vi "Periodic String Filter2.vi"(0 "Input String":string, 1 "reset?":bool, 2 "State":T1, 5 "Parameter":string, 9 "Remove Immediately?(F)":bool, 11 "Settings":T2={"threashold(#/s)"=1.0, "Check Peroid(s)"=1.0}, 12 "Exceeding processing capacity(F)":bool) -> (4 "Input String(dup)":string, 6 "oper":string, 8 ">> String-Parameter Map >>":variant=variant("CSM Tiny.DAQ: Break Continuous"=variant(u32 953145328), "CSM Tiny.DAQ: Close"=variant(u32 953145328), "CSM Tiny.DAQ: Configure"=variant(u32 953126122), "CSM Tiny.DAQ: Continuous Check"=variant(u32 953144928), "CSM Tiny.DAQ: Initialize"=variant(u32 953126122), "CSM Tiny.DAQ: Start"=variant(u32 953126122), "CSM Tiny.DAQ: Stop"=variant(u32 953145328), "CSM Tiny.Data"=variant(u32 953144928), "CSM Tiny.Data: Acquisite"=variant(u32 953144928), "CSM Tiny.UI: Refresh Buttons"=variant(u32 953145328)), 10 "Filtered Status":T3[](array[typedef]), 13 "Info":string[](array[string]), 14 "removed info":T3[](array[typedef]), 15 "filtered?":bool)   [LabVIEW 2017]
uses:
  user.lib/_NEVSTOP/Communicable State Machine(CSM)/Utility/Periodic String Filter Info.ctl
  user.lib/_NEVSTOP/Communicable State Machine(CSM)/Utility/Periodic String Filter State.ctl
  user.lib/_NEVSTOP/Communicable State Machine(CSM)/Communicable State Machine.lvlib
panel:
  out ">> Log Last Update Timestamp Map >>":variant=variant("CSM Tiny.DAQ: Break Continuous"=variant(u32 953145328), "CSM Tiny.DAQ: Close"=variant(u32 953145328), "CSM Tiny.DAQ: Configure"=variant(u32 953126122), "CSM Tiny.DAQ: Continuous Check"=variant(u32 953144928), "CSM Tiny.DAQ: Initialize"=variant(u32 953126122), "CSM Tiny.DAQ: Start"=variant(u32 953126122), "CSM Tiny.DAQ: Stop"=variant(u32 953145328), "CSM Tiny.Data"=variant(u32 953144928), "CSM Tiny.Data: Acquisite"=variant(u32 953144928), "CSM Tiny.UI: Refresh Buttons"=variant(u32 953145328))
  out ">> Log Count Map >>":variant=variant("CSM Tiny.DAQ: Break Continuous"=variant(i64 1), "CSM Tiny.DAQ: Close"=variant(i64 1), "CSM Tiny.DAQ: Configure"=variant(i64 1), "CSM Tiny.DAQ: Continuous Check"=variant(i64 192), "CSM Tiny.DAQ: Initialize"=variant(i64 1), "CSM Tiny.DAQ: Start"=variant(i64 1), "CSM Tiny.DAQ: Stop"=variant(i64 1), "CSM Tiny.Data"=variant(i64 97), "CSM Tiny.Data: Acquisite"=variant(i64 97), "CSM Tiny.UI: Refresh Buttons"=variant(i64 3))
  out ">> Log Last Check Count Map >>":variant=variant("CSM Tiny.DAQ: Break Continuous"=variant(i64 1), "CSM Tiny.DAQ: Close"=variant(i64 1), "CSM Tiny.DAQ: Configure"=variant(i64 1), "CSM Tiny.DAQ: Continuous Check"=variant(i64 188), "CSM Tiny.DAQ: Initialize"=variant(i64 1), "CSM Tiny.DAQ: Start"=variant(i64 1), "CSM Tiny.DAQ: Stop"=variant(i64 1), "CSM Tiny.Data"=variant(i64 95), "CSM Tiny.Data: Acquisite"=variant(i64 95), "CSM Tiny.UI: Refresh Buttons"=variant(i64 2))
  out ">> Log Last Check Timestamp Map >>":variant=variant("CSM Tiny.DAQ: Break Continuous"=variant(u32 953145328), "CSM Tiny.DAQ: Close"=variant(u32 953145328), "CSM Tiny.DAQ: Configure"=variant(u32 953126122), "CSM Tiny.DAQ: Continuous Check"=variant(u32 953144928), "CSM Tiny.DAQ: Initialize"=variant(u32 953126122), "CSM Tiny.DAQ: Start"=variant(u32 953126122), "CSM Tiny.DAQ: Stop"=variant(u32 953145328), "CSM Tiny.Data"=variant(u32 953144928), "CSM Tiny.Data: Acquisite"=variant(u32 953144928), "CSM Tiny.UI: Refresh Buttons"=variant(u32 953145328))
  out ">> Filtered Log Count Map >>":variant=variant("CSM Tiny.DAQ: Break Continuous"=variant(i64 1), "CSM Tiny.DAQ: Close"=variant(i64 1), "CSM Tiny.DAQ: Configure"=variant(i64 1), "CSM Tiny.DAQ: Continuous Check"=variant(i64 188), "CSM Tiny.DAQ: Initialize"=variant(i64 1), "CSM Tiny.DAQ: Start"=variant(i64 1), "CSM Tiny.DAQ: Stop"=variant(i64 1), "CSM Tiny.Data"=variant(i64 95), "CSM Tiny.Data: Acquisite"=variant(i64 95), "CSM Tiny.UI: Refresh Buttons"=variant(i64 2))
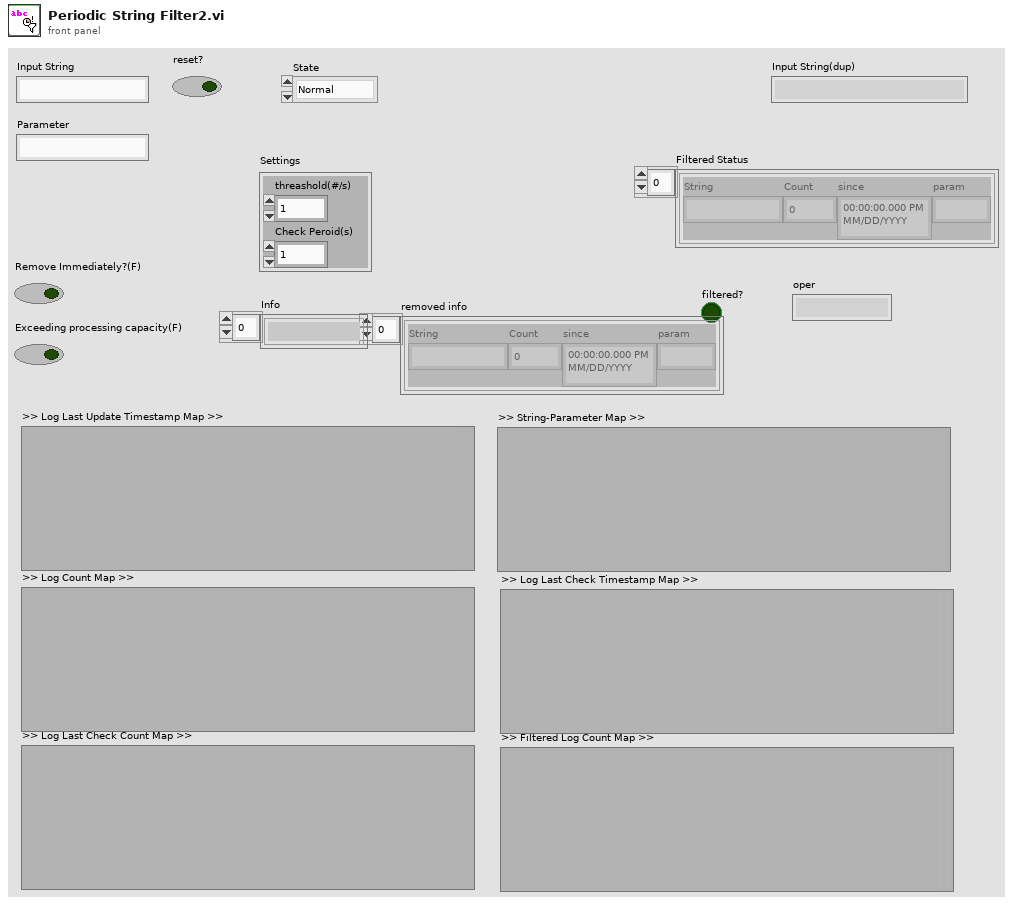
[diagram p1: front panel]
types:
  T1 = typedef "Communicable State Machine.lvlib/Periodic String Filter State.ctl" = enum16{"Normal", "Remove All Filters"}
  T2 = cluster{"threashold(#/s)":dbl, "Check Peroid(s)":dbl}
  T3 = typedef "Communicable State Machine.lvlib/Periodic String Filter Info.ctl" = cluster{"String":string, "Count":i64, "since":timestamp, "param":string}
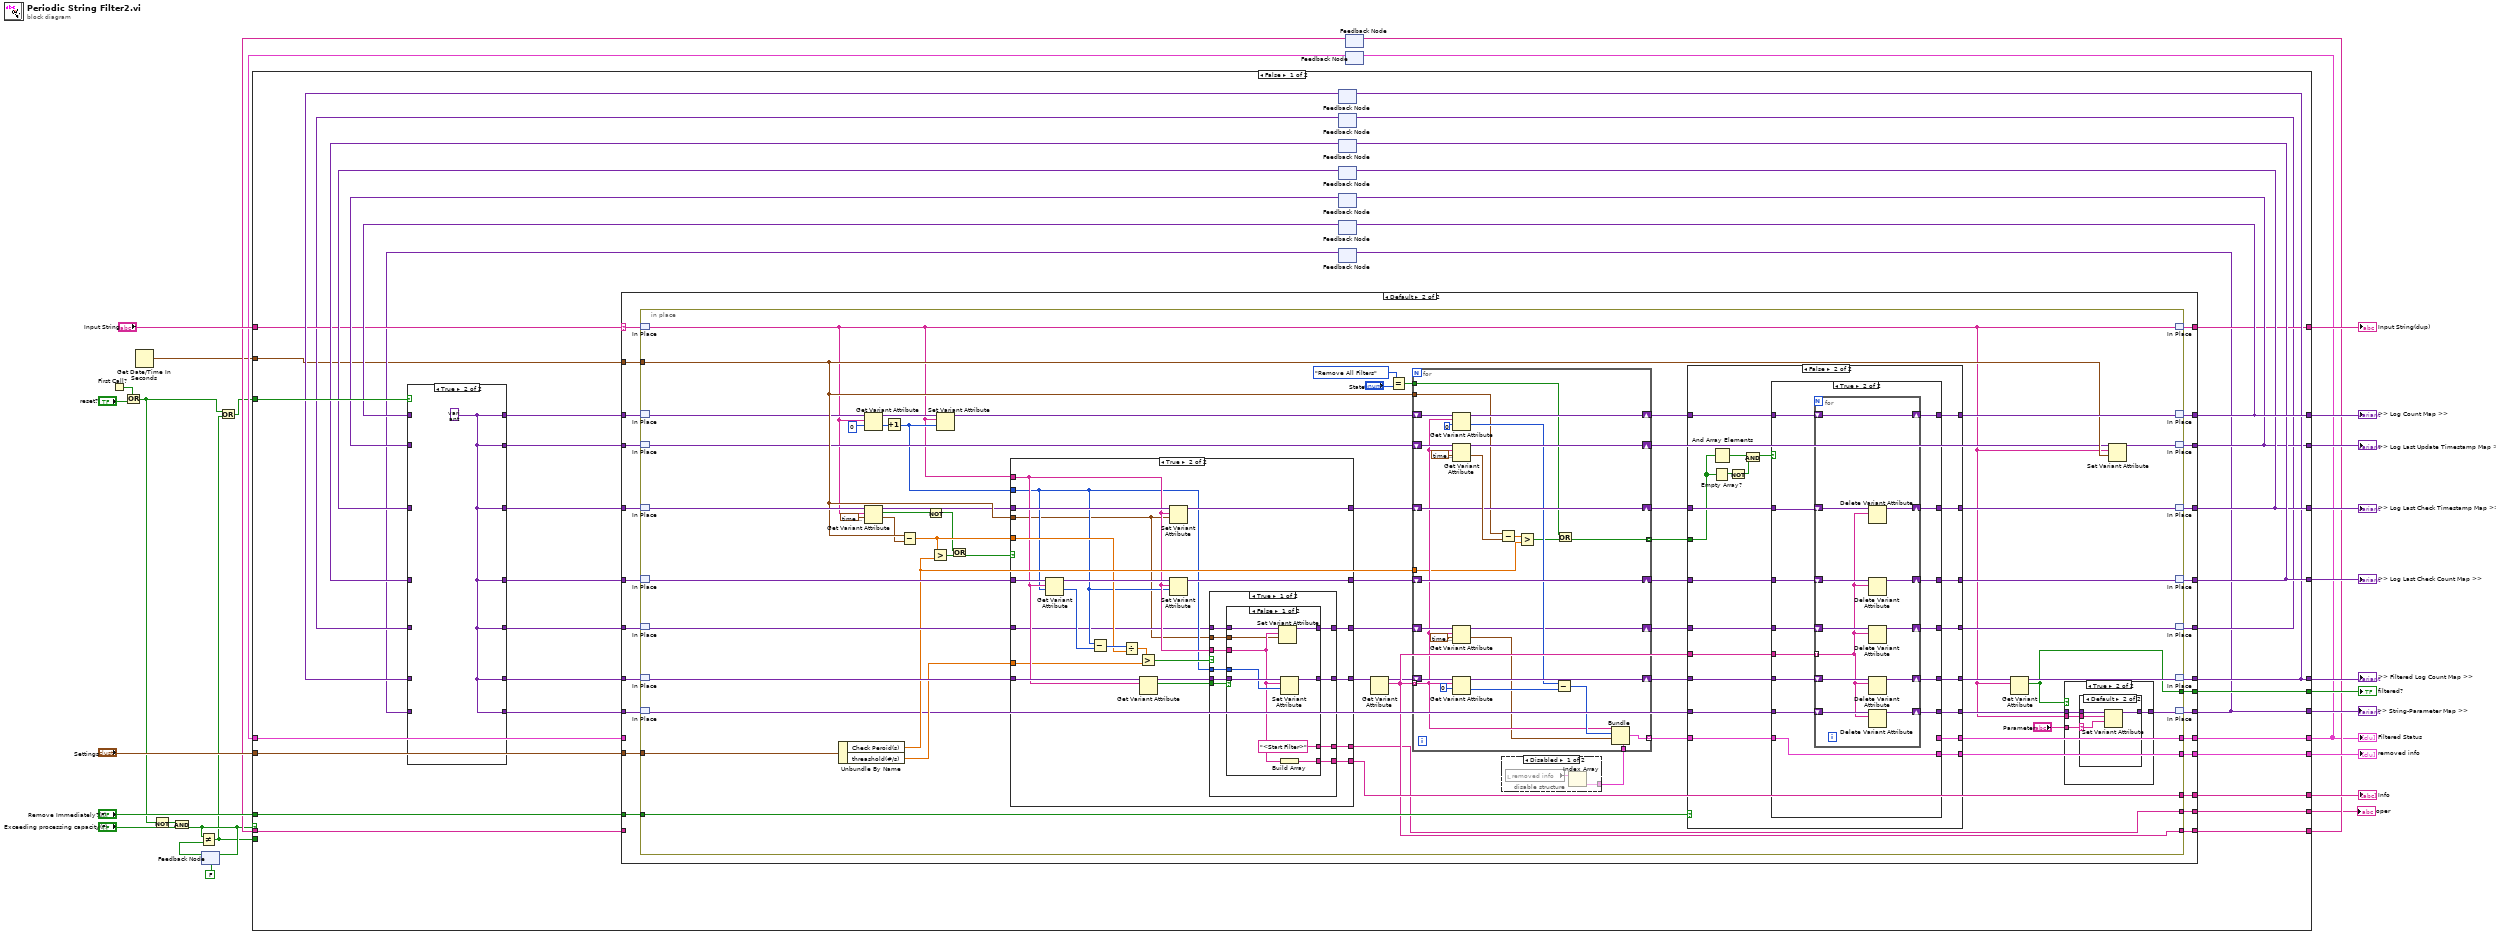
[diagram p0: block diagram]
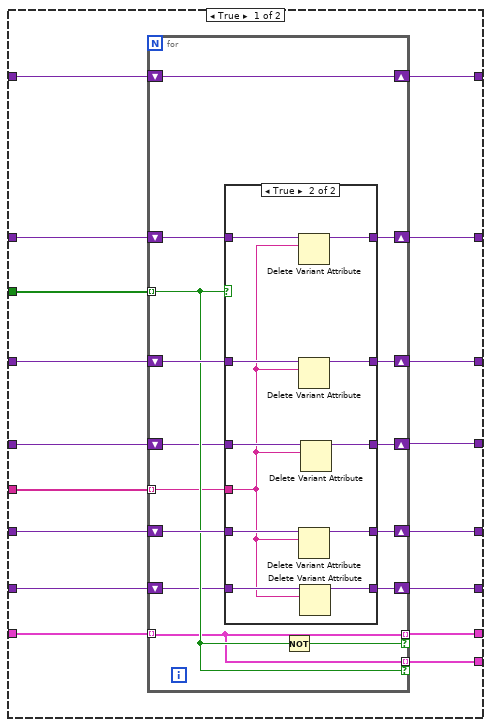
[diagram p5: hidden frame]
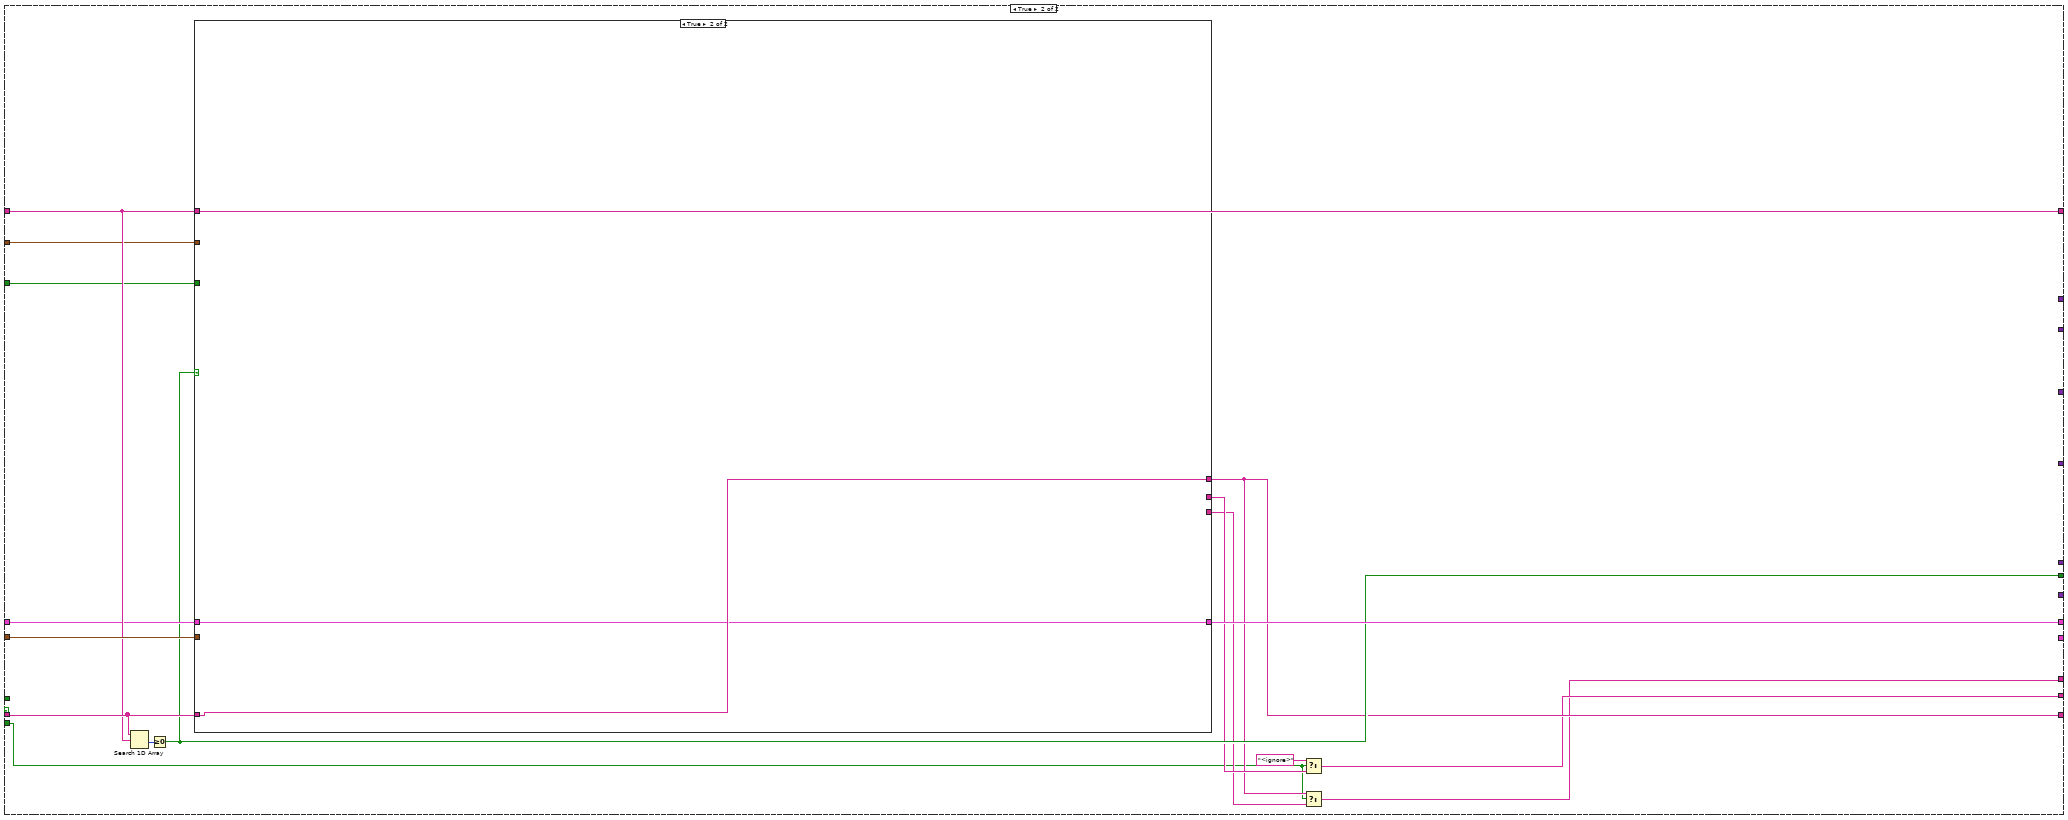
[diagram p13: hidden frame]
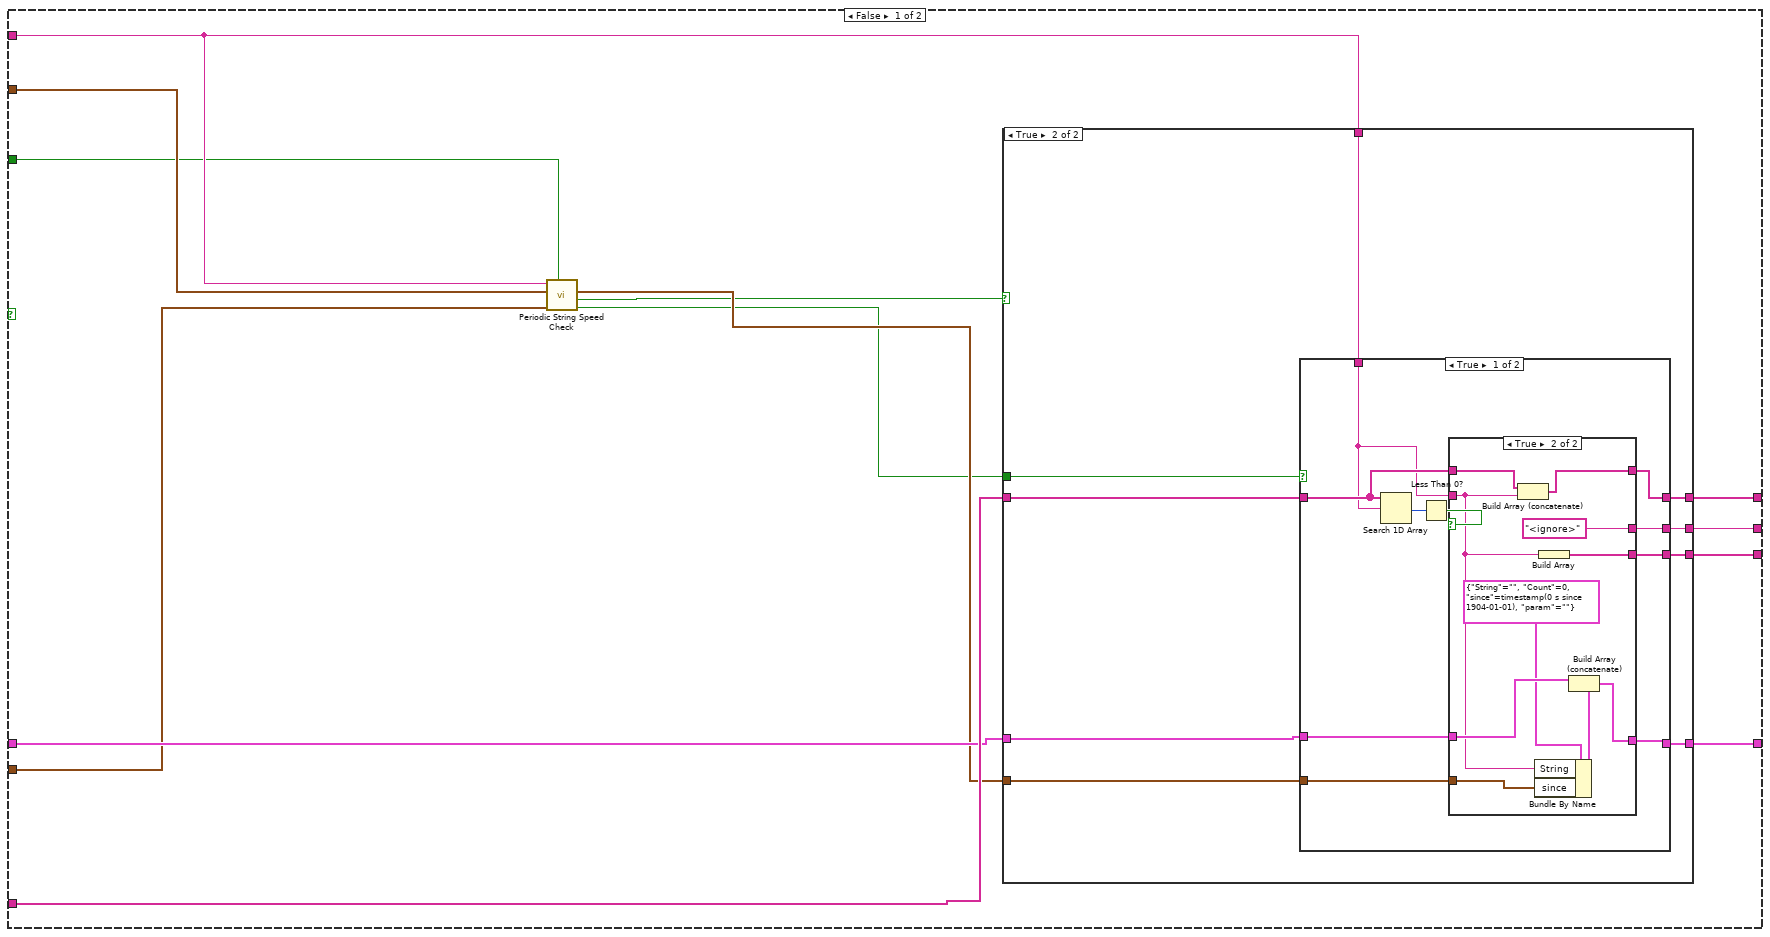
[diagram p14: hidden frame]
diagram:
  n1 = First Call?() -> (First Call?: T/F=w25:bool)
  n2 = Or(x=w25, y="reset?") -> (x .or. y?=w3:bool)
  n3 = Get Date/Time In Seconds() -> (seconds since 1Jan1904=w9:timestamp)
  n4 = Not(x=w3) -> (.not. x?=w7:bool)
  n5 = And(x=w7, y="Exceeding processing capacity(F)") -> (x .and. y?=w4:bool)
  n6 = feedback #1(FALSE) -> (w5:bool)
  n7 = Not Equal?(x=w4, y=w5) -> (x != y?=w1:bool)
  n8 = feedback-in #1(w4) -> ()
  n9 = Or(x=w3, y=w1) -> (x .or. y?=w2:bool)
  n10 = feedback #2() -> (w13:string[])  [unwired: 1 in]
  n11 = feedback #3() -> (w10:T3[])  [unwired: 1 in]
  n12 = case shown="False" w4 {
    tunnel: [w64 _] -> w29
    tunnel: [w63 _] -> w28
    tunnel: [w62 _] -> w27
    tunnel: [w61 w366] -> w26
    tunnel: w2 -> [w60 w364]
    tunnel: [w49 _] -> w23
    tunnel: [w48 _] -> w22
    tunnel: "Input String" -> [w47 w369]
    tunnel: [w46 w369] -> w20
    tunnel: [w45 _] -> w19
    tunnel: [w44 w357] -> w18
    tunnel: "Remove Immediately?(F)" -> [w43 _]
    tunnel: [w39 w367] -> w11
    tunnel: "Settings" -> [w38 w371]
    tunnel: [w35 _] -> w15
    tunnel: [w34 w360] -> w14
    tunnel: w13 -> [w33 w370]
    tunnel: w10 -> [w32 w368]
    tunnel: w9 -> [w31 w365]
    tunnel: [w30 w358] -> w8
    tunnel: w1 -> [_ w359]
    frame False {
      n13 = feedback #4() -> (w56:variant)  [unwired: 1 in]
      n14 = feedback #5() -> (w41:variant)  [unwired: 1 in]
      n15 = feedback #6() -> (w53:variant)  [unwired: 1 in]
      n16 = feedback #7() -> (w55:variant)  [unwired: 1 in]
      n17 = feedback #8() -> (w50:variant)  [unwired: 1 in]
      n18 = feedback #9() -> (w58:variant)  [unwired: 1 in]
      n19 = feedback #10() -> (w36:variant)  [unwired: 1 in]
      n20 = case shown="True" w60 {
        tunnel: [w355 w356] -> w59
        tunnel: w58 -> [w355 _]
        tunnel: [w350 w356] -> w57
        tunnel: w56 -> [w350 _]
        tunnel: w55 -> [w353 _]
        tunnel: [w353 w356] -> w54
        tunnel: w53 -> [w352 _]
        tunnel: [w352 w356] -> w52
        tunnel: [w354 w356] -> w51
        tunnel: w50 -> [w354 _]
        tunnel: [w351 w356] -> w42
        tunnel: w41 -> [w351 _]
        tunnel: [w349 w356] -> w37
        tunnel: w36 -> [w349 _]
        frame False {
        }
        frame True {
          w356 = variant
        }
      }
      n21 = case shown="Default" w47 {
        selector: w47 -> [_ w87]
        tunnel: [w73 w98] -> w64
        tunnel: [w70 w97] -> w63
        tunnel: [w71 w96] -> w62
        tunnel: [_ w95] -> w61
        tunnel: w59 -> [w73 w94]
        tunnel: w57 -> [w68 w93]
        tunnel: w54 -> [w71 w92]
        tunnel: w52 -> [w70 w91]
        tunnel: w51 -> [w72 w90]
        tunnel: [w68 w89] -> w49
        tunnel: [w72 w88] -> w48
        tunnel: [_ w86] -> w46
        tunnel: [w67 w85] -> w39
        tunnel: [_ w84] -> w45
        tunnel: [_ w83] -> w44
        tunnel: w43 -> [_ w82]
        tunnel: w31 -> [_ w81]
        tunnel: w42 -> [w69 w80]
        tunnel: [w69 w79] -> w40
        tunnel: w32 -> [w67 _]
        tunnel: w38 -> [_ w78]
        tunnel: w37 -> [w66 w77]
        tunnel: [w66 w76] -> w35
        tunnel: [w65 w75] -> w34
        tunnel: w33 -> [w65 _]
        tunnel: [_ w74] -> w30
        frame "" {
        }
        frame Default {
          n22 = in-place {
            in-place-border: [w139] -> w95
            in-place-border: [w148] -> w85
            in-place-border: [w149] -> w84
            in-place-border: [w153] -> w83
            in-place-border: w82 -> [w136]
            in-place-border: w81 -> [w147]
            in-place-border: w78 -> [w144]
            in-place-border: [w135] -> w75
            in-place-border: [w99] -> w74
            n23 = in-place-match #11(w87) -> (w100:string)
            n24 = in-place-match #12(w94) -> (w101:variant)
            n25 = in-place-match #13(w90) -> (w142:variant)
            n26 = in-place-match #14(w92) -> (w157:variant)
            n27 = in-place-match #15(w91) -> (w156:variant)
            n28 = in-place-match #16(w80) -> (w146:variant)
            n29 = in-place-match #17(w93) -> (w155:variant)
            n30 = in-place-match #18(w77) -> (w138:variant)
            n31 = Unbundle By Name(w144) -> ("Check Peroid(s)"=w140:dbl, "threashold(#/s)"=w143:dbl)
            n32 = Get Variant Attribute(Variant=w101, name=w100, default value (empty Variant)=i64 0 ("64bit integer")) -> (duplicate Variant=w132:variant, value=w133:i64)  [unwired: 1 in, 2 out]
            n33 = Get Variant Attribute(Variant=w157, name=w100, default value (empty Variant)=timestamp(0 s since 1904-01-01) ("current time")) -> (duplicate Variant=w131:variant, found=w125:bool, value=w130:timestamp)  [unwired: 1 in, 1 out]
            n34 = Increment(x=w133) -> (x+1=w129:i64)
            n35 = Subtract(x=w147, y=w130) -> (x-y=w128:dbl)
            n36 = Not(x=w125) -> (.not. x?=w124:bool)
            n37 = Greater?(x=w128, y=w140) -> (0:w127:bool)
            n38 = Set Variant Attribute(Variant=w132, name=w100, value=w129) -> (Variant out=w121:variant)  [unwired: 1 in, 2 out]
            n39 = Or(x=w124, y=w127) -> (x .or. y?=w126:bool)
            n40 = case shown="True" w126 {
              tunnel: w131 -> [w303 w325]
              tunnel: [w303 w324] -> w123
              tunnel: w147 -> [_ w307]
              tunnel: w156 -> [w302 w322]
              tunnel: [w302 w323] -> w122
              tunnel: w129 -> [_ w311]
              tunnel: w100 -> [_ w312]
              tunnel: w155 -> [w301 w314]
              tunnel: [w301 w319] -> w117
              tunnel: w128 -> [_ w315]
              tunnel: [_ w310] -> w153
              tunnel: w146 -> [w300 w309]
              tunnel: [w300 w308] -> w119
              tunnel: w143 -> [_ w306]
              tunnel: [_ w304] -> w99
              frame False {
              }
              frame True {
                n41 = Get Variant Attribute(Variant=w322, name=w312, default value (empty Variant)=w311) -> (duplicate Variant=w321:variant, value=w320:i64)  [unwired: 1 in, 2 out]
                n42 = Subtract(x=w311, y=w320) -> (x-y=w317:i64)
                n43 = Divide(x=w317, y=w315) -> (x/y=w316:dbl)
                n44 = Greater?(x=w316, y=w306) -> (0:w318:bool)
                n45 = Get Variant Attribute(Variant=w314, name=w312) -> (duplicate Variant=w313:variant, found=w305:bool)  [unwired: 2 in, 2 out]
                n46 = Set Variant Attribute(Variant=w325, name=w312, value=w307) -> (Variant out=w324:variant)  [unwired: 1 in, 2 out]
                n47 = Set Variant Attribute(Variant=w321, name=w312, value=w311) -> (Variant out=w323:variant)  [unwired: 1 in, 2 out]
                n48 = case shown="True" w318 {
                  tunnel: w313 -> [w332 w348]
                  tunnel: [w335 w348] -> w319
                  tunnel: w312 -> [w333 _]
                  tunnel: w311 -> [w334 _]
                  tunnel: w305 -> [w331 _]
                  tunnel: [w330 _] -> w310
                  tunnel: w309 -> [w329 w347]
                  tunnel: [w328 w347] -> w308
                  tunnel: w307 -> [w327 _]
                  tunnel: [w326 _] -> w304
                  frame True {
                    n49 = case shown="False" w331 {
                      tunnel: [w343 w346] -> w335
                      tunnel: w332 -> [w344 w346]
                      tunnel: w333 -> [w338 _]
                      tunnel: w334 -> [w342 _]
                      tunnel: [w341 _] -> w330
                      tunnel: w329 -> [w340 w345]
                      tunnel: [w339 w345] -> w328
                      tunnel: w327 -> [w337 _]
                      tunnel: ["<Start Filter>" ("Current State") _] -> w326
                      frame False {
                        n50 = Set Variant Attribute(Variant=w340, name=w338, value=w337) -> (Variant out=w339:variant)  [unwired: 1 in, 2 out]
                        n51 = Set Variant Attribute(Variant=w344, name=w338, value=w342) -> (Variant out=w343:variant)  [unwired: 1 in, 2 out]
                        n52 = Build Array(w338) -> (w341:string[])
                      }
                      frame True {
                      }
                    }
                  }
                  frame False {
                  }
                }
              }
            }
            n53 = Get Variant Attribute(Variant=w117) -> (duplicate Variant=w102:variant, names=w135:string[])  [unwired: 3 in, 2 out]
            n54 = Equal?(x=Periodic_String_Filter_State."Remove All Filters", y="State") -> (x = y?=w105:bool)
            n55 = disable-structure shown="Disabled" {
              disable-tunnel: [w270 _] -> w108
              frame Disabled {
                n56 = local read "removed info"() -> (w271:T3[])
                n57 = Index Array(array=w271) -> (element=w270:T3)  [unwired: 1 in]
              }
              frame Enabled {
              }
            }
            n58 = for {
              tunnel: w135 -> [w278] mode=indexing
              shift-right: [w289] -> w113
              shift-left: w102 -> [w296]
              shift-right: [w297] -> w115
              shift-left: w122 -> [w297]
              shift-right: [w291] -> w116
              shift-left: w123 -> [w291]
              shift-right: [w292] -> w118
              shift-left: w142 -> [w293]
              shift-right: [w290] -> w112
              shift-left: w121 -> [w295]
              tunnel: [w283] -> w110 mode=indexing
              tunnel: [w273] -> w111 mode=indexing
              tunnel: w147 -> [w281]
              shift-right: [w276] -> w109
              shift-left: w119 -> [w280]
              tunnel: w140 -> [w275]
              tunnel: w108 -> [w274]
              tunnel: w105 -> [w272]
              n59 = Get Variant Attribute(Variant=w295, name=w278, default value (empty Variant)=i64 0) -> (duplicate Variant=w290:variant, value=w285:i64)  [unwired: 1 in, 2 out]
              n60 = Get Variant Attribute(Variant=w293, name=w278, default value (empty Variant)=timestamp(0 s since 1904-01-01) ("current time")) -> (duplicate Variant=w292:variant, value=w294:timestamp)  [unwired: 1 in, 2 out]
              n61 = Get Variant Attribute(Variant=w280, name=w278, default value (empty Variant)=timestamp(0 s since 1904-01-01) ("current time")) -> (duplicate Variant=w276:variant, value=w277:timestamp)  [unwired: 1 in, 2 out]
              n62 = Get Variant Attribute(Variant=w296, name=w278, default value (empty Variant)=i64 0) -> (duplicate Variant=w289:variant, value=w286:i64)  [unwired: 1 in, 2 out]
              n63 = Subtract(x=w281, y=w294) -> (x-y=w298:dbl)
              n64 = Greater?(x=w298, y=w275) -> (0:w282:bool)
              n65 = Subtract(x=w285, y=w286) -> (x-y=w284:i64)
              n66 = Or(x=w272, y=w282) -> (x .or. y?=w273:bool)
              n67 = Bundle(cluster=w274, "String"=w278, "Count"=w284, "since"=w277) -> (w283:T3)  [unwired: 1 in]
            }
            n68 = case shown="False" w136 {
              tunnel: [w184 w236] -> w152
              tunnel: w116 -> [w183 w235]
              tunnel: [w182 w234] -> w151
              tunnel: w115 -> [w181 w233]
              tunnel: [w180 w232] -> w114
              tunnel: w113 -> [w176 w231]
              tunnel: w112 -> [w179 w226]
              tunnel: [w178 w225] -> w150
              tunnel: [w177 w224] -> w149
              tunnel: w111 -> [w174 w223]
              tunnel: w135 -> [w175 w222]
              tunnel: [w173 w221] -> w148
              tunnel: w110 -> [w170 w220]
              tunnel: w109 -> [w172 w219]
              tunnel: [w171 w218] -> w145
              tunnel: w138 -> [w168 w217]
              tunnel: [w169 w216] -> w104
              frame True {
                n69 = for {
                  shift-right: [w198] -> w184
                  shift-left: w183 -> [w199]
                  shift-right: [w196] -> w182
                  shift-left: w181 -> [w197]
                  shift-right: [w195] -> w180
                  shift-left: w176 -> [w193]
                  tunnel: w175 -> [w188] mode=indexing
                  shift-right: [w194] -> w178
                  shift-left: w179 -> [w194]
                  tunnel: [w187] -> w177 mode=indexing if=w192
                  tunnel: w174 -> [w192] mode=indexing
                  tunnel: [w187] -> w173 mode=indexing if=w191
                  shift-right: [w190] -> w171
                  shift-left: w172 -> [w189]
                  tunnel: w170 -> [w187] mode=indexing
                  shift-right: [w186] -> w169
                  shift-left: w168 -> [w185]
                  n70 = case shown="True" w192 {
                    tunnel: w199 -> [w204 w215]
                    tunnel: [w204 w214] -> w198
                    tunnel: w197 -> [w203 w213]
                    tunnel: [w203 w212] -> w196
                    tunnel: [w202 w211] -> w195
                    tunnel: w188 -> [_ w205]
                    tunnel: w193 -> [w202 w210]
                    tunnel: [w201 w209] -> w190
                    tunnel: w189 -> [w201 w208]
                    tunnel: [w200 w207] -> w186
                    tunnel: w185 -> [w200 w206]
                    frame False {
                    }
                    frame True {
                      n71 = Delete Variant Attribute(6:w205, 7:w215) -> (3:w214:variant)  [unwired: 1 in, 2 out]
                      n72 = Delete Variant Attribute(6:w205, 7:w213) -> (3:w212:variant)  [unwired: 1 in, 2 out]
                      n73 = Delete Variant Attribute(6:w205, 7:w210) -> (3:w211:variant)  [unwired: 1 in, 2 out]
                      n74 = Delete Variant Attribute(6:w205, 7:w206) -> (3:w207:variant)  [unwired: 1 in, 2 out]
                      n75 = Delete Variant Attribute(6:w205, 7:w208) -> (3:w209:variant)  [unwired: 1 in, 2 out]
                    }
                  }
                  n76 = Not(x=w192) -> (.not. x?=w191:bool)
                }
              }
              frame False {
                n77 = Empty Array?(array=w223) -> (empty?=w228:bool)
                n78 = And Array Elements(Boolean array=w223) -> (logical AND=w229:bool)
                n79 = Not(x=w228) -> (.not. x?=w227:bool)
                n80 = And(x=w229, y=w227) -> (x .and. y?=w230:bool)
                n81 = case shown="True" w230 {
                  tunnel: [w243 w256] -> w236
                  tunnel: w235 -> [w243 w257]
                  tunnel: [w242 w254] -> w234
                  tunnel: w233 -> [w242 w255]
                  tunnel: [w241 w253] -> w232
                  tunnel: w231 -> [w241 w250]
                  tunnel: w226 -> [w240 w252]
                  tunnel: [w240 w251] -> w225
                  tunnel: [_ w246] -> w224
                  tunnel: w222 -> [_ w249]
                  tunnel: [w239 _] -> w221
                  tunnel: w220 -> [w239 w246]
                  tunnel: w219 -> [w238 w248]
                  tunnel: [w238 w247] -> w218
                  tunnel: w217 -> [w237 w245]
                  tunnel: [w237 w244] -> w216
                  frame False {
                  }
                  frame True {
                    n82 = for {
                      shift-right: [w268] -> w256
                      shift-left: w257 -> [w269]
                      shift-right: [w266] -> w254
                      shift-left: w255 -> [w267]
                      shift-right: [w265] -> w253
                      shift-left: w250 -> [w263]
                      tunnel: w249 -> [w258] mode=indexing
                      shift-right: [w264] -> w251
                      shift-left: w252 -> [w264]
                      shift-right: [w262] -> w247
                      shift-left: w248 -> [w261]
                      shift-right: [w259] -> w244
                      shift-left: w245 -> [w260]
                      n83 = Delete Variant Attribute(6:w258, 7:w269) -> (3:w268:variant)  [unwired: 1 in, 2 out]
                      n84 = Delete Variant Attribute(6:w258, 7:w267) -> (3:w266:variant)  [unwired: 1 in, 2 out]
                      n85 = Delete Variant Attribute(6:w258, 7:w261) -> (3:w262:variant)  [unwired: 1 in, 2 out]
                      n86 = Delete Variant Attribute(6:w258, 7:w263) -> (3:w265:variant)  [unwired: 1 in, 2 out]
                      n87 = Delete Variant Attribute(6:w258, 7:w260) -> (3:w259:variant)  [unwired: 1 in, 2 out]
                    }
                  }
                }
              }
            }
            n88 = Get Variant Attribute(Variant=w114, name=w100) -> (duplicate Variant=w154:variant, found=w139:bool)  [unwired: 2 in, 2 out]
            n89 = case shown="True" w139 {
              tunnel: w104 -> [w158 w162]
              tunnel: w100 -> [_ w161]
              tunnel: [w158 w160] -> w137
              tunnel: "Parameter" -> [_ w159]
              frame False {
              }
              frame True {
                n90 = case shown="Default" w159 {
                  selector: w159 -> [_ w164]
                  tunnel: w162 -> [w163 w167]
                  tunnel: w161 -> [_ w166]
                  tunnel: [w163 w165] -> w160
                  frame "" {
                  }
                  frame Default {
                    n91 = Set Variant Attribute(Variant=w167, name=w166, value=w164) -> (Variant out=w165:variant)  [unwired: 1 in, 2 out]
                  }
                }
              }
            }
            n92 = Set Variant Attribute(Variant=w118, name=w100, value=w147) -> (Variant out=w141:variant)  [unwired: 1 in, 2 out]
            n93 = in-place-match #11(w100) -> (w86:string)
            n94 = in-place-match #12(w150) -> (w98:variant)
            n95 = in-place-match #13(w141) -> (w88:variant)
            n96 = in-place-match #14(w152) -> (w96:variant)
            n97 = in-place-match #15(w151) -> (w97:variant)
            n98 = in-place-match #16(w145) -> (w79:variant)
            n99 = in-place-match #17(w154) -> (w89:variant)
            n100 = in-place-match #18(w137) -> (w76:variant)
          }
        }
      }
      n101 = feedback-in #4(w49) -> ()
      n102 = feedback-in #5(w40) -> ()
      n103 = feedback-in #6(w63) -> ()
      n104 = feedback-in #7(w62) -> ()
      n105 = feedback-in #8(w48) -> ()
      n106 = feedback-in #9(w64) -> ()
      n107 = feedback-in #10(w35) -> ()
    }
    frame True {
      n108 = Search 1D Array(1D array=w370, element=w369) -> (index of element=w372:i32)  [unwired: 1 in]
      n109 = Greater Or Equal To 0?(x=w372) -> (x >= 0?=w366:bool)
      n110 = case shown="True" w366 {
        tunnel: w371 -> [w381 _]
        tunnel: w370 -> [w385 w422]
        tunnel: [w384 w422] -> w360
        tunnel: w369 -> [w380 _]
        tunnel: w368 -> [w383 w421]
        tunnel: [w382 w421] -> w367
        tunnel: w365 -> [w376 _]
        tunnel: [w375 _] -> w362
        tunnel: [w374 _] -> w361
        tunnel: w364 -> [w373 _]
        frame False {
          n111 = call "Periodic String Speed Check.vi"("reset?"=w373, "Settings"=w381, "seconds since 1Jan1904"=w376, "element"=w380) -> ("over threashold?"=w377:bool, "Peroid?"=w378:bool, "timestamp"=w379:timestamp)  [unwired: 4 in, 1 out]
          n112 = case shown="True" w378 {
            tunnel: w385 -> [w387 w396]
            tunnel: [w387 w395] -> w384
            tunnel: w380 -> [_ w394]
            tunnel: w383 -> [w386 w393]
            tunnel: [w386 w392] -> w382
            tunnel: w379 -> [_ w391]
            tunnel: w377 -> [_ w390]
            tunnel: [_ w389] -> w375
            tunnel: [_ w388] -> w374
            frame False {
            }
            frame True {
              n113 = case shown="True" w390 {
                tunnel: w396 -> [w404 w420]
                tunnel: [w403 w420] -> w395
                tunnel: w394 -> [w402 _]
                tunnel: w393 -> [w401 w419]
                tunnel: [w400 w419] -> w392
                tunnel: w391 -> [w399 _]
                tunnel: [w398 _] -> w389
                tunnel: [w397 _] -> w388
                frame True {
                  n114 = Search 1D Array(1D array=w404, element=w402) -> (index of element=w406:i32)  [unwired: 1 in]
                  n115 = Less Than 0?(x=w406) -> (x < 0?=w405:bool)
                  n116 = case shown="True" w405 {
                    tunnel: w404 -> [w408 w418]
                    tunnel: [w408 w417] -> w403
                    tunnel: w402 -> [_ w410]
                    tunnel: w401 -> [w407 w416]
                    tunnel: [w407 w415] -> w400
                    tunnel: w399 -> [_ w412]
                    tunnel: [_ "<ignore>" ("Current State")] -> w398
                    tunnel: [_ w409] -> w397
                    frame False {
                    }
                    frame True {
                      n117 = Build Array (concatenate)(w418, w410) -> (w417:string[])
                      n118 = Bundle By Name(cluster=T3 {"String"="", "Count"=0, "since"=timestamp(0 s since 1904-01-01), "param"=""} ("element"), "String"=w410, "since"=w412) -> (w413:T3)
                      n119 = Build Array(w410) -> (w409:string[])
                      n120 = Build Array (concatenate)(w416, w413) -> (w415:T3[])
                    }
                  }
                }
                frame False {
                }
              }
            }
          }
        }
        frame True {
        }
      }
      n121 = Select(t="<ignore>" ("Current State"), s=w359, f=w362) -> (s? t:f=w358:string)
      n122 = Select(t=w360, s=w359, f=w361) -> (s? t:f=w357:string[])
    }
  }
  ">> Log Count Map >>" <- w29
  ">> Log Last Check Timestamp Map >>" <- w27
  ">> Log Last Check Count Map >>" <- w28
  "filtered?" <- w26
  ">> Filtered Log Count Map >>" <- w23
  ">> Log Last Update Timestamp Map >>" <- w22
  "Input String(dup)" <- w20
  "Filtered Status" <- w11
  "removed info" <- w19
  "Info" <- w18
  ">> String-Parameter Map >>" <- w15
  "oper" <- w8
  n123 = feedback-in #2(w14) -> ()
  n124 = feedback-in #3(w11) -> ()
